vi "历史温度曲线.vi"() -> ()   [LabVIEW 2016, in "斯坦道CODcr.lvlib"]
uses:
  <vilib>/Utility/miscctls.llb/LVPointTypeDef.ctl
  <vilib>/Utility/tdmsutil.llb/TDMSFileViewerLocalizedText.vi
panel:
  out "名称":string
  in  "选项卡控件":enum32{"趋势图", "测试数据"}(tab)
  out "波形图":waveform(dbl)[](graph)
  out "显示值":string
  in  "多列列表框":i32(listbox)
  in  "列表框":i32(listbox)
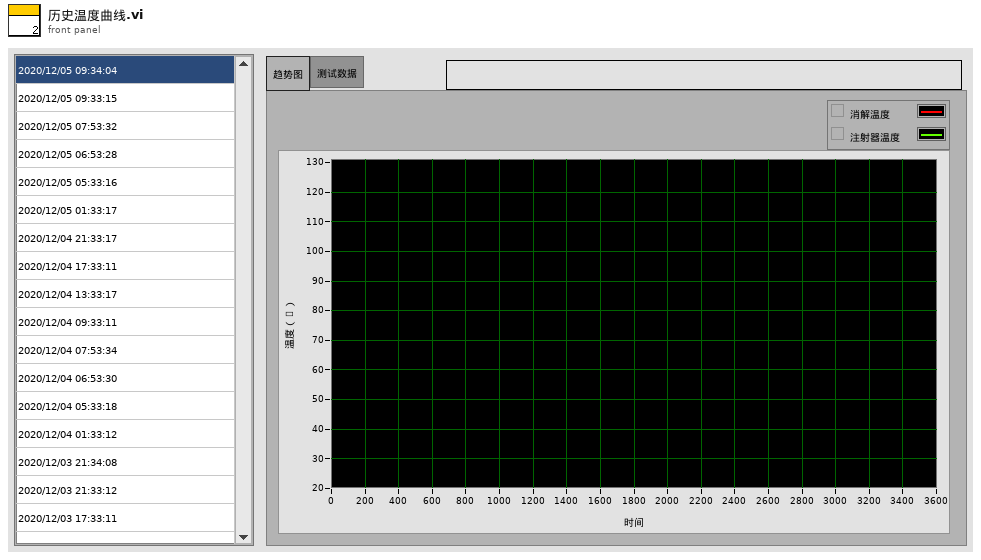
[diagram p1: front panel]
types:
  T1 = typedef "LVPointTypeDef.ctl" = cluster{"Horizontal":i16, "Vertical":i16}
  T2 = typedef "LVPoint32TypeDef.ctl" = cluster{"Horizontal":i32, "Vertical":i32}
  T3 = typedef "Type Enum.ctl" = enum8{"Void", "I8", "I16", "I32", "I64", "U8", "U16", "U32", "U64", "Single Float", "Double Float", "Extended Float", "Single Complex", "Double Complex", "Extended Complex", "Enum I8 NEVER", "Enum I16 NEVER", "Enum I32 NEVER", "Enum I64 NEVER", "Enum U8", "Enum U16", "Enum U32", "Enum U64", "Single Float With Unit", "Double Float With Unit", "Extended Float With Unit", "Single Complex With Unit", "Double Complex With Unit", "Extended Complex With Unit", "boolU16", "Boolean", "String", "Handle", "Path", "Picture", "C String", "Pascal String", "Tag", "SubString", "Array", "SubArray", "Cluster", "Numeric Cluster", "Variant", "LV Variant", "Measure Data (waveform)", "Refnum", "ExtData", "function", "Typedef", "Poly VI", "bad wire", "LabVIEW Class Instance"}
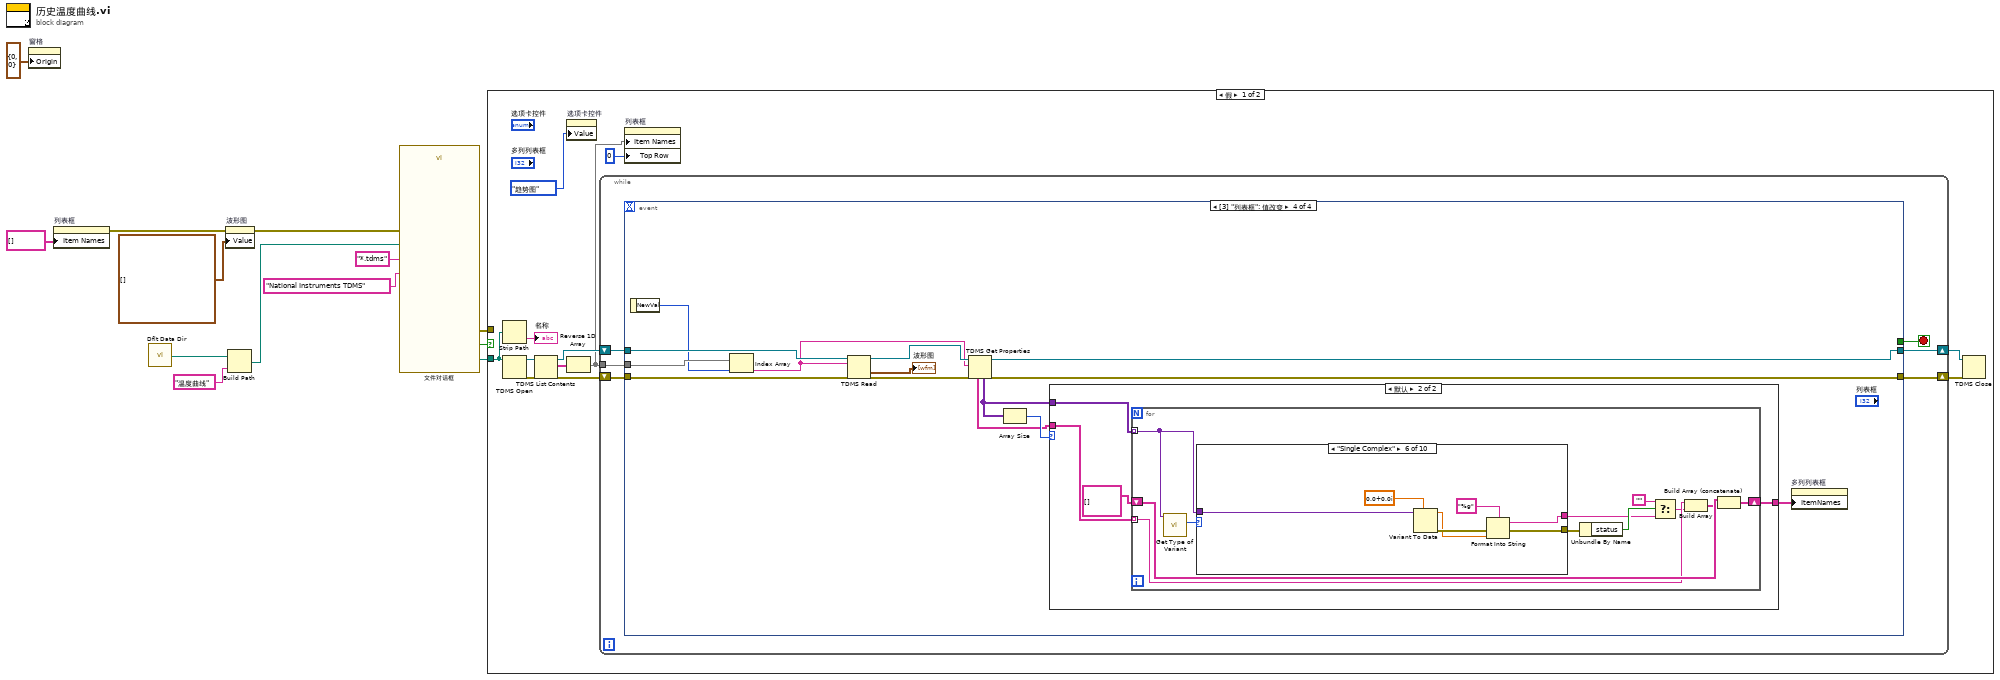
[diagram p0: block diagram]
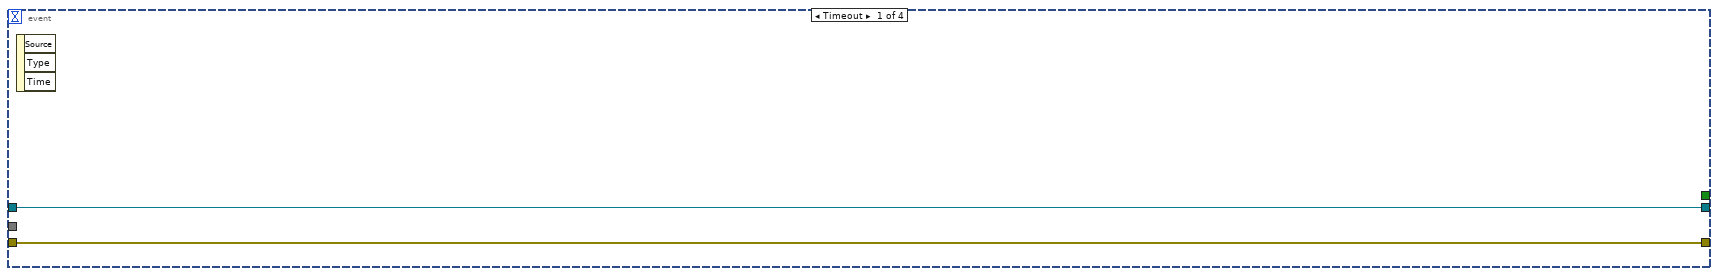
[diagram p2: hidden frame]
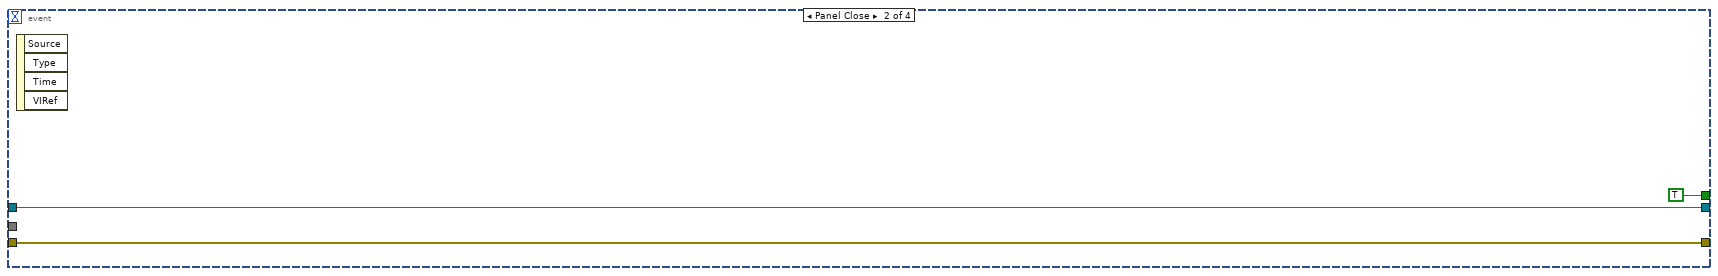
[diagram p3: hidden frame]
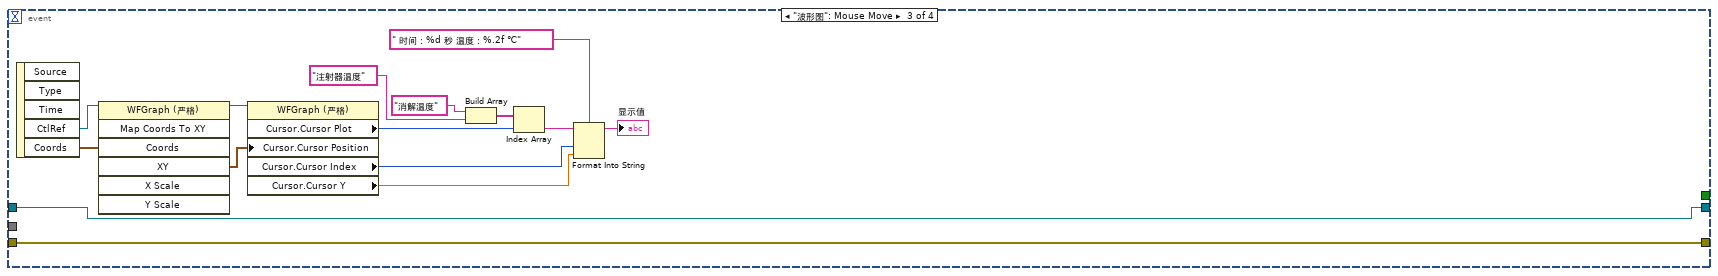
[diagram p4: hidden frame]
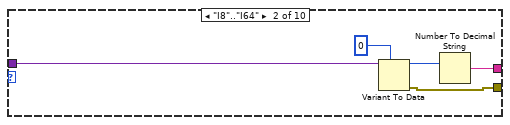
[diagram p7: hidden frame]
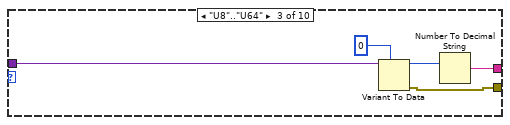
[diagram p8: hidden frame]
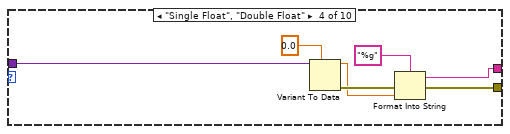
[diagram p9: hidden frame]
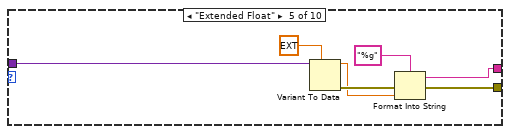
[diagram p10: hidden frame]
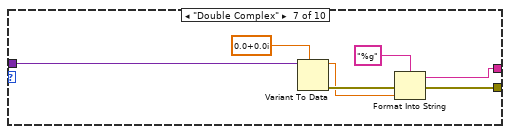
[diagram p11: hidden frame]
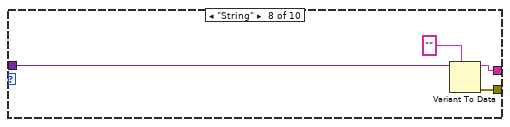
[diagram p12: hidden frame]
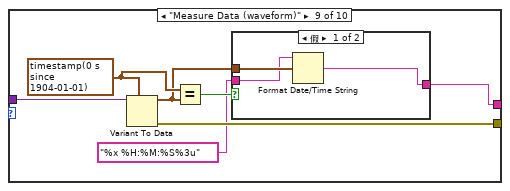
[diagram p13: hidden frame]
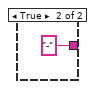
[diagram p14: hidden frame]
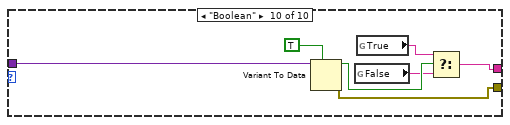
[diagram p15: hidden frame]
diagram:
  n1 = property on="窗格" class="Pane"("Origin"=T1 {"Horizontal"=0, "Vertical"=0} ("原点")) -> ()  [unwired: 2 in, 2 out]
  n2 = property on="列表框" class="LstBox (严格)"("Item Names"=string[] [] ("项名")) -> (error out=w2:errorcluster)  [unwired: 2 in, 1 out]
  n3 = call <vilib>:"Dflt Data Dir.vi"() -> ("App:Default Data Directory"=w9:path)
  n4 = property on="波形图" class="WFGraph (严格)"(error in=w2, "Value"=waveform(dbl)[] [] ("波形图")) -> (error out=w1:errorcluster)  [unwired: 1 in, 1 out]
  n5 = Build Path(base path=w9, name or relative path="温度曲线" ("名称或相对路径")) -> (appended path=w10:path)
  n6 = call "文件对话框"("start path"=w10, "error in"=w1, "pattern (all files)"="*.tdms", "pattern label"="National Instruments TDMS") -> ("selected path"=w11:path, "cancelled"=w7:bool, "error out"=w6:errorcluster)  [unwired: 8 in, 1 out]
  n7 = case shown="假" w7 {
    tunnel: w11 -> [w18 _]
    tunnel: w6 -> [_ _]
    frame False {
      n8 = Strip Path(path=w18) -> (name=→"名称":string)  [unwired: 1 out]
      n9 = TDMS Open(11:w18) -> (0:w22:errorcluster, 3:w25:refnum<k34>)  [unwired: 6 in]
      n10 = TDMS List Contents(4:w22, 7:w25) -> (0:w23:errorcluster, 2:w19:string[], 3:w24:refnum<k34>)  [unwired: 1 in, 1 out]
      n11 = property on="选项卡控件" class="TabCtl (严格)"("Value"=enum32{"趋势图", "测试数据"}."趋势图" ("选项卡控件")) -> ()  [unwired: 2 in, 2 out]
      n12 = Reverse 1D Array(array=w19) -> (reversed array=w14:string[])
      n13 = while {
        tunnel: w14 -> [w27]
        shift-right: [w29] -> w21
        shift-left: w24 -> [w31]
        shift-right: [w28] -> w20
        shift-left: w23 -> [w30]
        stop <- w26 stop-if-true
        n14 = event shown="[3] \"列表框\": 值改变" {
          selector: _ -> [_ _ _ _]
          dyn-events: _ -> [_ _ _ _]
          timeout: _ -> [_ _ _ _]
          tunnel: w31 -> [w33 w35 w48 w65]
          tunnel: w30 -> [w32 w34 w47 w64]
          tunnel: [w33 w35 w48 w54] -> w29
          tunnel: [w32 w34 w47 w53] -> w28
          tunnel: w27 -> [_ _ _ w63]
          tunnel: [_ TRUE _ _] -> w26
          event Timeout {
            n15 = event-data() -> ()  [unwired: 1 in, 3 out]
          }
          event Panel Close {
            n16 = event-data() -> ()  [unwired: 1 in, 4 out]
          }
          event "波形图": Mouse Move {
            n17 = event-data() -> ("CtlRef"=w46:refnum<vi>, "Coords"=w45:T2)  [unwired: 1 in, 3 out]
            n18 = invoke on="调用节点" class="WFGraph (严格)" method="Map Coords To XY"(reference=w46, "Coords"=w45) -> (reference out=w43:refnum<vi>, "XY"=w51:cluster{"X":dbl, "Y":dbl})  [unwired: 5 in, 5 out]
            n19 = property on="属性节点" class="WFGraph (严格)"(reference=w43, "Cursor.Cursor Position"=w51) -> ("Cursor.Cursor Plot"=w41:i32, "Cursor.Cursor Index"=w49:i32, "Cursor.Cursor Y"=w42:dbl)  [unwired: 1 in, 2 out]
            n20 = Build Array("消解温度", "注射器温度") -> (w38:string[])
            n21 = Index Array(array=w38, index=w41) -> (element=w37:string)
            n22 = Format Into String(format string=" 时间：%d 秒 温度：%.2f ℃" ("格式字符串"), initial string=w37, w49, w42) -> (resulting string=→"显示值":string)  [unwired: 1 in, 1 out]
          }
          event "列表框": Value Change {
            n23 = event-data() -> ("NewVal"=w62:i32)  [unwired: 1 in]
            n24 = Index Array(array=w63, index=w62) -> (element=w56:string)
            n25 = TDMS Read(0:w65, 5:w56, 11:w64) -> (4:w57:refnum<k34>, 10:→"波形图":waveform(dbl)[], 15:w55:errorcluster)  [unwired: 5 in, 3 out]
            n26 = TDMS Get Properties(8:w55, 10:w56, 11:w57) -> (0:w53:errorcluster, 3:w54:refnum<k34>, 4:w58:variant[], 6:w59:string[])  [unwired: 3 in, 2 out]
            n27 = Array Size(array=w58) -> (size(s)=w60:i32)
            n28 = case shown="默认" w60 {
              tunnel: w59 -> [_ w69]
              tunnel: w58 -> [_ w68]
              tunnel: [_ w66] -> w52
              frame 0 {
              }
              frame Default {
                n29 = for {
                  tunnel: w68 -> [w80] mode=indexing
                  tunnel: w69 -> [w77] mode=indexing
                  shift-right: [w78] -> w66
                  shift-left: string[][] [] -> [w79]
                  n30 = call <vilib>:"Get Type of Variant.vi"("Data In"=w80) -> ("Type Enum"=w76:T3)  [unwired: 9 in, 1 out]
                  n31 = case shown="\"Single Complex\"" w76 {
                    tunnel: w80 -> [_ w85 w90 w97 w104 w111 w118 w122 w129 w140]
                    tunnel: [_ w82 w87 w94 w100 w107 w115 w120 w128 w139] -> w75
                    tunnel: [_ w81 w86 w93 w99 w108 w114 w119 w127 w136] -> w73
                    frame "Void", Default {
                    }
                    frame "I8".."I64" {
                      n32 = Variant To Data(type=i64 0 ("offset (0)"), Variant=w85) -> (data=w83:i64, error out=w82:errorcluster)  [unwired: 1 in]
                      n33 = Number To Decimal String(number=w83) -> (decimal integer string=w81:string)  [unwired: 1 in]
                    }
                    frame "U8".."U64" {
                      n34 = Variant To Data(type=u64 0 ("offset (0)"), Variant=w90) -> (data=w88:u64, error out=w87:errorcluster)  [unwired: 1 in]
                      n35 = Number To Decimal String(number=w88) -> (decimal integer string=w86:string)  [unwired: 1 in]
                    }
                    frame "Single Float", "Double Float" {
                      n36 = Variant To Data(type=0.0 ("offset (0)"), Variant=w97) -> (data=w91:dbl, error out=w95:errorcluster)  [unwired: 1 in]
                      n37 = Format Into String(format string="%g", error in=w95, w91) -> (resulting string=w93:string, error out=w94:errorcluster)  [unwired: 1 in]
                    }
                    frame "Extended Float" {
                      n38 = Variant To Data(type=ext 0.0 ("offset (0)"), Variant=w104) -> (data=w98:ext, error out=w101:errorcluster)  [unwired: 1 in]
                      n39 = Format Into String(format string="%g", error in=w101, w98) -> (resulting string=w99:string, error out=w100:errorcluster)  [unwired: 1 in]
                    }
                    frame "Single Complex" {
                      n40 = Variant To Data(type=csg 0.0+0.0i, Variant=w111) -> (data=w106:csg, error out=w109:errorcluster)  [unwired: 1 in]
                      n41 = Format Into String(format string="%g", error in=w109, w106) -> (resulting string=w108:string, error out=w107:errorcluster)  [unwired: 1 in]
                    }
                    frame "Double Complex" {
                      n42 = Variant To Data(type=cdb 0.0+0.0i, Variant=w118) -> (data=w113:cdb, error out=w116:errorcluster)  [unwired: 1 in]
                      n43 = Format Into String(format string="%g", error in=w116, w113) -> (resulting string=w114:string, error out=w115:errorcluster)  [unwired: 1 in]
                    }
                    frame "String" {
                      n44 = Variant To Data(type="" ("offset (0)"), Variant=w122) -> (data=w119:string, error out=w120:errorcluster)  [unwired: 1 in]
                    }
                    frame "Measure Data (waveform)" {
                      w126 = timestamp(0 s since 1904-01-01) ("offset (0)")
                      n45 = Variant To Data(type=w126, Variant=w129) -> (data=w125:timestamp, error out=w128:errorcluster)  [unwired: 1 in]
                      n46 = Equal?(x=w126, y=w125) -> (x = y?=w124:bool)
                      n47 = case shown="假" w124 {
                        tunnel: w125 -> [w132 _]
                        tunnel: [w131 "-" ("date/time string")] -> w127
                        tunnel: "%x %H:%M:%S%3u" ("time format string (%c)") -> [w130 _]
                        frame False {
                          n48 = Format Date/Time String(time format string (%c)=w130, seconds (now)=w132) -> (date/time string=w131:string)  [unwired: 1 in]
                        }
                        frame True {
                        }
                      }
                    }
                    frame "Boolean" {
                      n49 = Variant To Data(type=TRUE, Variant=w140) -> (data=w137:bool, error out=w139:errorcluster)  [unwired: 1 in]
                      n50 = global read "TDMSFileViewerLocalizedText.vi" "False"() -> (w135:string)
                      n51 = global read "TDMSFileViewerLocalizedText.vi" "True"() -> (w134:string)
                      n52 = Select(t=w134, s=w137, f=w135) -> (s? t:f=w136:string)
                    }
                  }
                  n53 = Unbundle By Name(w75) -> ("status"=w74:bool)
                  n54 = Select(t="", s=w74, f=w73) -> (s? t:f=w71:string)
                  n55 = Build Array(w77, w71) -> (w70:string[])
                  n56 = Build Array (concatenate)(w79, w70) -> (w78:string[][])
                }
              }
            }
            n57 = property on="多列列表框" class="MCListbox (严格)"("ItemNames"=w52) -> ()  [unwired: 2 in, 2 out]
          }
        }
      }
      n58 = property on="列表框" class="LstBox (严格)"("Item Names"=w14, "Top Row"=0 ("顶行")) -> ()  [unwired: 2 in, 2 out]
      n59 = TDMS Close(8:w20, 11:w21) -> ()  [unwired: 2 out]
    }
    frame True {
    }
  }
